vi "process.vi"(8 "error in (no error)":errorcluster, 11 "MQTT_Base in":refnum<class "MQTT_Base.lvclass">) -> ()   [LabVIEW 2013, in "MQTT Server.lvlib" / "MQTT_Base.lvclass"]
uses:
  MQTT_Base.lvclass
  MQTT_Base.lvclass/MQTT_Base.ctl
panel:
  out "class name":string
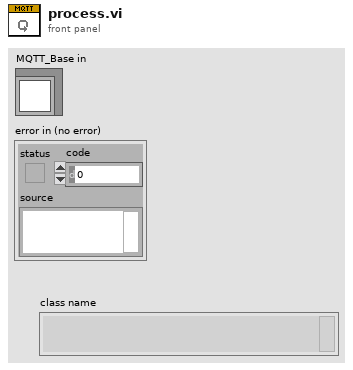
[diagram p1: front panel]
types:
  T1 = typedef "MQTT Server.lvlib/MQTT_Base.lvclass/Response -- cluster.ctl" = cluster{"Packet":refnum<class "ControlPacket.lvclass">, "Protocol Error":errorcluster, "disconnect session":bool, "[ACK]":refnum<notifier>[]}
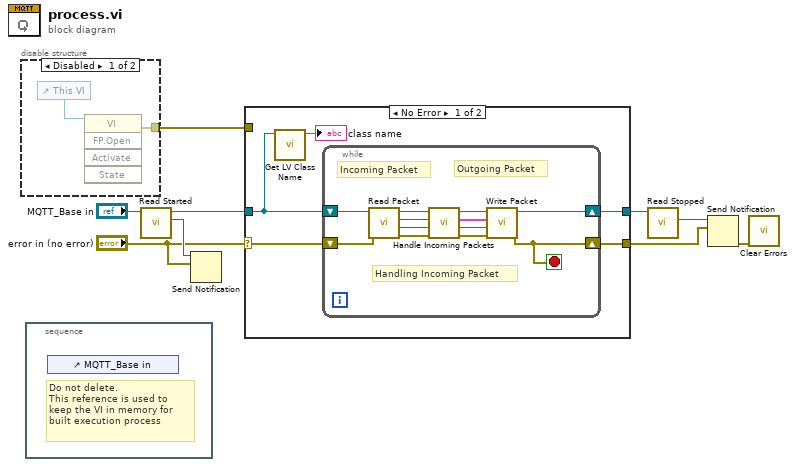
[diagram p0: block diagram]
diagram:
  n1 = disable-structure shown="Disabled" {
    disable-tunnel: [w10 _] -> w1
    frame Disabled {
      n2 = control-ref of="This VI"() -> (w11:refnum<vi>)
      n3 = invoke class="VI" method="FP.Open"(reference=w11) -> (error out=w10:errorcluster)  [unwired: 4 in, 4 out]
    }
    frame Enabled {
    }
  }
  n4 = stacked-sequence {
    frame #0 {
      # "Do not delete.\nThis reference is used to keep the VI in memory for built execution process"
      n5 = control-ref of="MQTT_Base in"() -> ()  [unwired: 1 out]
    }
  }
  n6 = call "Read Started.vi"("MQTT_Base in"="MQTT_Base in") -> ("Started"=w5:refnum<notifier>, "MQTT_Base out"=w3:refnum<class "MQTT_Base.lvclass">)  [unwired: 8 in, 1 out]
  n7 = Send Notification(notification="error in (no error)", notifier=w5) -> ()  [unwired: 1 in, 2 out]
  n8 = case shown="No Error" "error in (no error)" {
    selector: "error in (no error)" -> [w13 w30]
    tunnel: [w16 w30] -> w7
    tunnel: [w15 w29] -> w9
    tunnel: w3 -> [w12 w29]
    tunnel: w1 -> [_ _]
    frame No Error {
      n9 = call <vilib>:"Get LV Class Name.vi"("object"=w12) -> ("class name"=→"class name":string)  [unwired: 9 in, 1 out]
      n10 = while {
        shift-right: [w25] -> w15
        shift-left: w12 -> [w28]
        shift-right: [w17] -> w16
        shift-left: w13 -> [w18]
        stop <- w17 stop-if-true
        # "Handling Incoming Packet"
        # "Outgoing Packet"
        # "Incoming Packet"
        n11 = call "Read Packet.vi"("error in (no error)"=w18, "MQTT_Base in"=w28) -> ("error out"=w19:errorcluster, "SessionMailbox"=w21:refnum<queue>, "Packet"=w22:refnum<class "ControlPacket.lvclass">, "MQTT_Base out"=w27:refnum<class "MQTT_Base.lvclass">)  [unwired: 6 in]
        n12 = call-dynamic "Handle Incoming Packets.vi"("error in (no error)"=w19, "SessionMailbox"=w21, "Incoming Packet"=w22, "MQTT_Base in"=w27) -> ("error out"=w24:errorcluster, "SessionMailbox out"=w20:refnum<queue>, "Outgoing"=w23:T1, "MQTT_Base out"=w26:refnum<class "MQTT_Base.lvclass">)  [unwired: 4 in]
        n13 = call "Write Packet.vi"("error in (no error)"=w24, "SessionMailbox in"=w20, "Outgoing"=w23, "MQTT_Base in"=w26) -> ("error out"=w17:errorcluster, "MQTT_Base out"=w25:refnum<class "MQTT_Base.lvclass">)  [unwired: 6 in]
      }
    }
    frame Error {
    }
  }
  n14 = call "Read Stopped.vi"("MQTT_Base in"=w9) -> ("Stopped"=w8:refnum<notifier>)  [unwired: 8 in, 2 out]
  n15 = Send Notification(notification=w7, notifier=w8) -> (error out=w6:errorcluster)  [unwired: 1 in, 1 out]
  n16 = call <vilib>:"Clear Errors.vi"("error in (no error)"=w6) -> ()  [unwired: 6 in, 1 out]
